vi "close.vi"(8 "error in (no error)":errorcluster, 11 "midiPlayer in":refnum<class "midiPlayer.lvclass">) -> (0 "error out":errorcluster, 3 "midiPlayer out":refnum<class "midiPlayer.lvclass">)   [LabVIEW 2020, in "midiPlayer.lvclass"]
uses:
  midiPlayer.lvclass
  midiPlayer.lvclass/midiPlayer.ctl
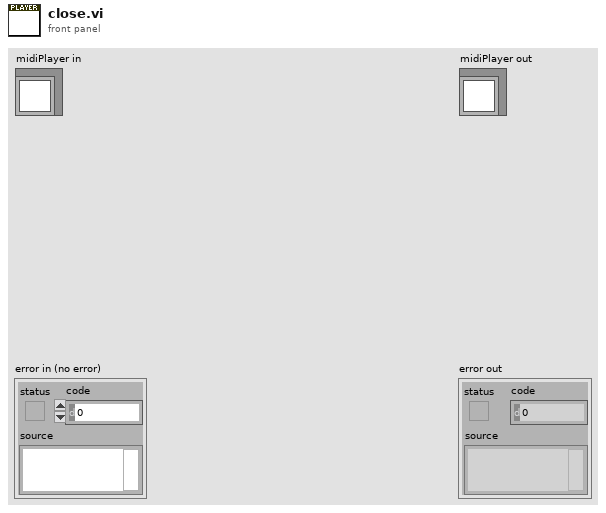
[diagram p1: front panel]
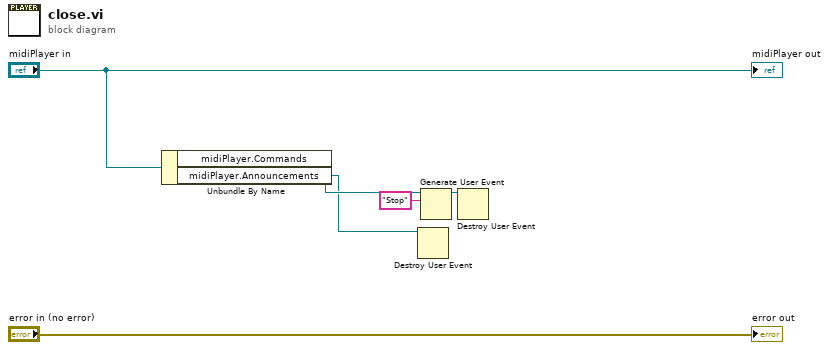
[diagram p0: block diagram]
diagram:
  n1 = Unbundle By Name("midiPlayer in") -> ("midiPlayer.Commands"=w4:refnum<user-event>, "midiPlayer.Announcements"=w3:refnum<user-event>)
  n2 = Destroy User Event(user event=w3) -> ()  [unwired: 1 in, 1 out]
  n3 = Generate User Event(user event=w4, event data cluster="Stop" ("event data")) -> (user event out=w6:refnum<user-event>)  [unwired: 2 in, 1 out]
  n4 = Destroy User Event(user event=w6) -> ()  [unwired: 1 in, 1 out]
  "error out" <- "error in (no error)"
  "midiPlayer out" <- "midiPlayer in"
